vi "AddCondiments.vi"(8 "error in (no error)":errorcluster, 11 "Tea in":refnum<class "Tea.lvclass">) -> (0 "error out":errorcluster, 2 "ProcessMessage":string, 3 "Tea out":refnum<class "Tea.lvclass">)   [LabVIEW 2013, in "Tea.lvclass"]
uses:
  Tea.lvclass
  CaffeineBeverage.lvclass/CaffeineBeverage.lvclass
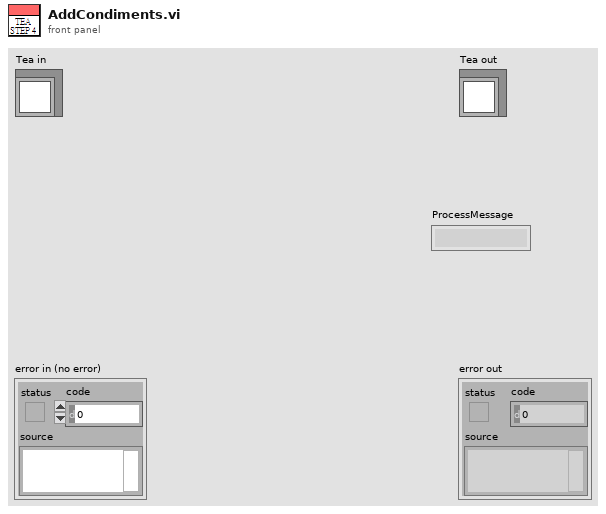
[diagram p1: front panel]
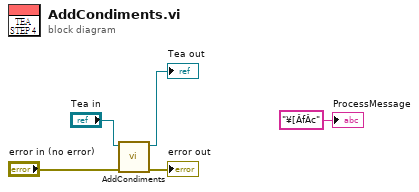
[diagram p0: block diagram]
diagram:
  n1 = call-parent "AddCondiments.vi"("error in (no error)"="error in (no error)", "CaffeineBeverage in"="Tea in") -> ("error out"=→"error out":errorcluster, "CaffeineBeverage out"=→"Tea out":refnum<class "Tea.lvclass">)  [unwired: 7 in, 1 out]
  "ProcessMessage" <- "¥[ÂfÂc" ("ProcessMessage")
